vi "Load Configuration File.vi"(8 "error in (no error)":errorcluster, 10 "Filename":string="XC-(18-05-2020)-HG-ITR-500us_13598.xca", 11 "Bobcat 640 in":refnum<class "Bobcat 640.lvclass">) -> (0 "error out":errorcluster, 3 "Bobcat 640 out":refnum<class "Bobcat 640.lvclass">)   [LabVIEW 2018, in "Bobcat 640.lvlib" / "Bobcat 640.lvclass"]
uses:
  Bobcat 640.lvclass
  Bobcat 640.lvclass/Bobcat 640.ctl
  <vilib>/vision/driver/NI_Vision_Acquisition_Software.lvlib
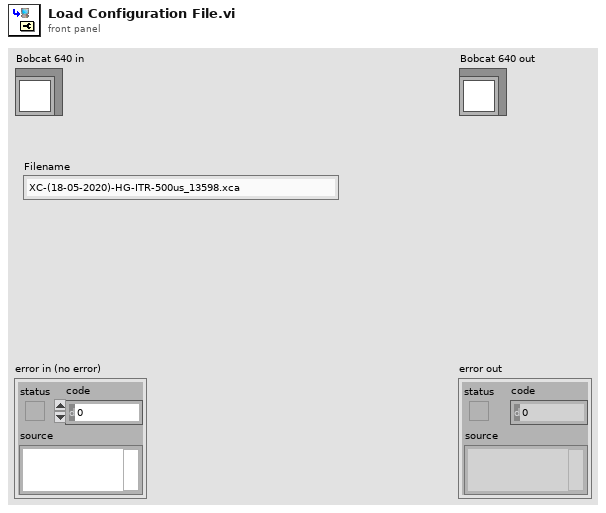
[diagram p1: front panel]
types:
  T1 = typedef "IMAQdx.ctl" = refnum<k21>
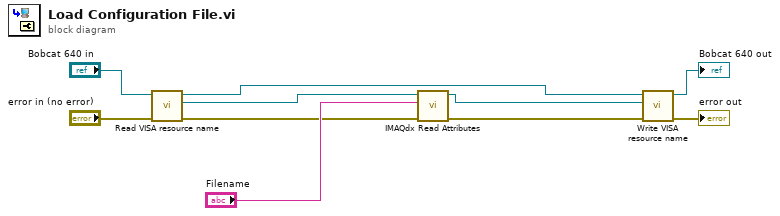
[diagram p0: block diagram]
diagram:
  n1 = call "Read VISA resource name.vi"("error in (no error)"="error in (no error)", "Bobcat 640 in"="Bobcat 640 in") -> ("error out"=w3:errorcluster, "IMAQdx Session"=w5:T1, "Bobcat 640 out"=w6:refnum<class "Bobcat 640.lvclass">)  [unwired: 7 in]
  n2 = call <vilib>:"IMAQdx Read Attributes.vi"("error in"=w3, "Filename"="Filename", "Session In"=w5) -> ("error out"=w2:errorcluster, "Session Out"=w1:T1)  [unwired: 7 in]
  n3 = call "Write VISA resource name.vi"("error in (no error)"=w2, "IMAQdx Session"=w1, "Bobcat 640 in"=w6) -> ("error out"=→"error out":errorcluster, "Bobcat 640 out"=→"Bobcat 640 out":refnum<class "Bobcat 640.lvclass">)  [unwired: 7 in]
